vi "GameToIAStateOffensive.vi"(8 "error in (no error)":errorcluster, 11 "Game in":refnum<class "Game.lvclass">) -> (0 "error out":errorcluster, 1 "RobotRef":refnum<class "Robot.lvclass">[](array[class]), 2 "IA State out":T1={"our_robots"=[], "enemy_robots"=[], "balls"=[], "geometry"={"line_width"=0, "field_length"=0, "field_width"=0, "boundary_width"=0, "referee_width"=0, "goal_width"=0, "goal_depth"=0, "goal_wall_width"=0, "center_circle_radius"=0, "defense_radius"=0, "defense_stretch"=0, "free_kick_from_defense_dist"=0, "penalty_spot_from_field_line_dist"=0, "penalty_line_from_spot_dist"=0}, "IA Judge"={"stage"="", "command"="", "our_goalie_id"=0.0, "enemy_goalie_id"=0.0, "command enum"=enum."Halt", "Time"=enum."Azul"}, "Received Timestamp"=timestamp(0 s since 1904-01-01), "Events"={"Touch"=FALSE, "Ball out"=FALSE, "id touch"=0.0, "Ball out of \nVision"=FALSE, "Ball inside \nGoalie area"=FALSE, "Robot not responding"=FALSE, "Robots responding status"=[1.0, 1.0, 1.0, 1.0, 1.0, 1.0], "Enemy Ball \nPossession"=FALSE, "Pass State"=FALSE, "id end of pass"=0.0, "Kick"=FALSE, "Id ini Possession"=0.0, "Ball Possesion"=FALSE, "Id Possesion"=0.0, "Direct Kick"=FALSE, "2nd Strk Ativo"=FALSE}}, 3 "Game out":refnum<class "Game.lvclass">, 4 "Parameters.lvclass":refnum<class "Parameters.lvclass">)   [LabVIEW 2023, in "Game.lvclass"]
uses:
  Game.lvclass
  Vision_class/Old vision/SSL Detection Frame Simple Estimator Cameras VelCmd Folder/Core/AI Input.ctl
  Vision_class/Old vision/Controls/AI Robot.ctl
  Vision_class/Old vision/Controls/Functions Enum.ctl
  Vision_class/Old vision/Controls/AttackerStates.ctl
  Vision_class/Old vision/Controls/PathDests.ctl
  Vision_class/Old vision/Controls/PathDest.ctl
  Navigation/VSSNavigation/VSSAttackerStates.ctl
  Vision_class/Old vision/SSL Detection Frame Simple Estimator Cameras VelCmd Folder/Core/AI Ball.ctl
  Vision_class/Old vision/SSL Detection Frame Simple Estimator Cameras VelCmd Folder/Core/Field Size.ctl
  Vision_class/Old vision/SSL Detection Frame Simple Estimator Cameras VelCmd Folder/Core/AI Judge.ctl
  Communication_class/Paths/MessageAI_State Folder/Intel/Command Enum.ctl
  Vision_class/Old vision/SSL Detection Frame Simple Estimator Cameras VelCmd Folder/Util/Events/Events.ctl
  Robot_class/Robot.lvclass
  Parameters_class/Parameters.lvclass
  Team_class/OffensivePlay.ctl
  Game.lvclass/Game.ctl
  Team_class/Team.lvclass/Team.ctl
  Object_class/Object.lvclass/Object.ctl
  Ball_class/Ball.lvclass/Ball.ctl
  Events_class/Events.lvclass/Events.ctl
  Referee_class/Referee.lvclass/Referee.ctl
  Robot_class/Robot.lvclass/Robot.ctl
  Robot_class/Read id.vi
  Object_class/Read x.vi
  Object_class/Read y.vi
  Robot_class/Read orientation.vi
  Robot_class/Read est_v_tang.vi
  Robot_class/Read est_v_norm.vi
  Object_class/Read pos_est_x.vi
  Object_class/Read pos_est_y.vi
  Robot_class/Read dribble.vi
  Robot_class/Read path.vi
  Robot_class/Read path_smooth.vi
  Robot_class/Read dest_x.vi
  Robot_class/Read dest_y.vi
  Robot_class/Read dest_orientation.vi
  Robot_class/Read role.vi
  Read Parameters.lvclass.vi
  Read OffensiveTeam.vi
  Read EnemyRef.vi
  Read BallRef.vi
  Read EventsRef.vi
  Read FieldRef.vi
  Read Referee.vi
  Read TimeRef.vi
  Referee_class/Read command_from_referee.vi
  Referee_class/Read command_interpreted.vi
  Events_class/Read ball_inside_enemy_goalie_area.vi
  Events_class/Read ball_inside_our_goalie_area.vi
  Events_class/Read ball_out.vi
  Events_class/Read ball_out_of_vision.vi
  Events_class/Read enemy_ball_possesion.vi
  Events_class/Read id_enemy_ball_possesion.vi
  Events_class/Read id_our_balll_possesion.vi
  Events_class/Read id_touch.vi
  Events_class/Read kick.vi
  Events_class/Read our_balll_possesion.vi
  Events_class/Read touch.vi
  Ball_class/Read v_x.vi
  Ball_class/Read v_y.vi
  Team_class/Read RobotRef.vi
  Team_class/Read OffensivePlay.vi
  Ball_class/Ball.lvclass
  Enemy_class/Enemy.lvclass
  Ally_class/Ally.lvclass
  Events_class/Events.lvclass
  Field_class/Field.lvclass
  Referee_class/Referee.lvclass
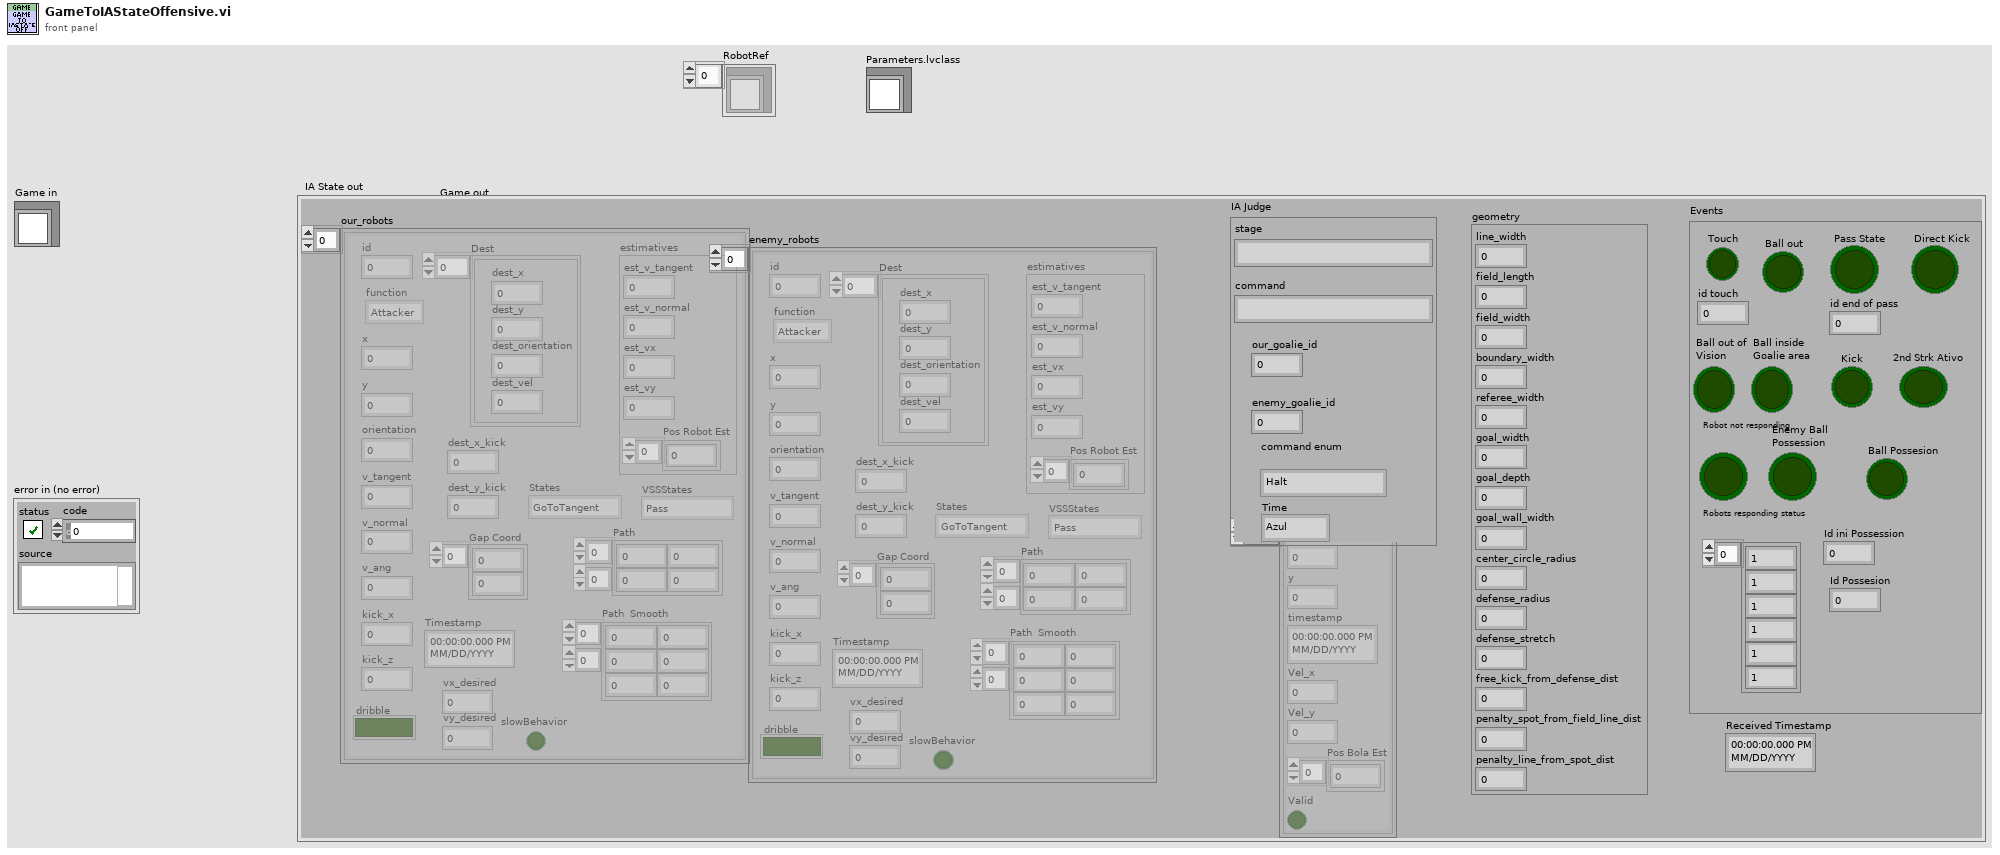
[diagram p1: front panel]
types:
  T1 = typedef "AI Input.ctl" = cluster{"our_robots":T2[], "enemy_robots":T2[], "balls":T8[], "geometry":T9, "IA Judge":T10, "Received Timestamp":timestamp, "Events":T12}
  T2 = typedef "AI Robot.ctl" = cluster{"id":u32, "function":T3, "x":dbl, "y":dbl, "orientation":dbl, "v_tangent":dbl, "v_normal":dbl, "v_ang":dbl, "kick_x":dbl, "kick_z":dbl, "dribble":bool, "Timestamp":timestamp, "estimatives":cluster{"est_v_tangent":dbl, "est_v_normal":dbl, "est_vx":dbl, "est_vy":dbl, "Pos Robot Est":dbl[]}, "dest_x_kick":dbl, "dest_y_kick":dbl, "Gap Coord":dbl[], "States":T4, "Path ":dbl[][], "Path  Smooth":dbl[][], "Dest":T5, "vx_desired":dbl, "vy_desired":dbl, "slowBehavior":bool, "VSSStates":T7}
  T3 = typedef "Functions Enum.ctl" = enum16{"2nd Striker", "Attacker", "Goalie", "Defender", "Striker", "Goto 0", "Dummy", "Kicker", "ZigZag 0", "ZigZag 1", "ZigZag 2", "ZigZag 3", "ZigZag 4", "ZigZag 5", "ZigZag 6", "ZigZag 7", "ZigZag 8", ""}
  T4 = typedef "AttackerStates.ctl" = enum16{"Pass", "GoToTangent", "BallGetting", "GoToKick", ""}
  T5 = typedef "PathDests.ctl" = T6[]
  T6 = typedef "PathDest.ctl" = cluster{"dest_x":dbl, "dest_y":dbl, "dest_orientation":dbl, "dest_vel":dbl}
  T7 = typedef "VSSAttackerStates.ctl" = enum16{"Pass", "GoToTangent", "BallGetting", "GoToKick", "Rotate anti-clockwise", "Rotate Clockwise", ""}
  T8 = typedef "AI Ball.ctl" = cluster{"x":dbl, "y":dbl, "timestamp":timestamp, "Vel_x":dbl, "Vel_y":dbl, "Pos Bola Est":dbl[], "Valid":bool}
  T9 = typedef "Field Size.ctl" = cluster{"line_width":u32, "field_length":u32, "field_width":u32, "boundary_width":u32, "referee_width":u32, "goal_width":u32, "goal_depth":u32, "goal_wall_width":u32, "center_circle_radius":u32, "defense_radius":u32, "defense_stretch":u32, "free_kick_from_defense_dist":u32, "penalty_spot_from_field_line_dist":u32, "penalty_line_from_spot_dist":u32}
  T10 = typedef "AI Judge.ctl" = cluster{"stage":string, "command":string, "our_goalie_id":dbl, "enemy_goalie_id":dbl, "command enum":T11, "Time":enum16{"Azul", "Amarelo"}}
  T11 = typedef "Command Enum.ctl" = enum16{"Halt", "Stop", "Force Start", "PKA Normal Start", "Prepare Kickoff Ally", "PKE Normal Start", "Prepare Kickoff Enemy", "Prepare Penalty Ally", "PPA Normal Start", "Prepare Penalty Enemy", "PPE Normal Start", "Direct Free Enemy", "Direct Free Ally", "Indirect Free Enemy", "Indirect Free Ally", "Timeout Enemy", "Timeout Ally", "Goal Enemy", "Goal Ally", "Ball Placement Enemy", "Ball Placement Ally", "Normal Half Time", "Extra Time Break", "Extra Half Time", "None", "Post Game"}
  T12 = typedef "Events.ctl" = cluster{"Touch":bool, "Ball out":bool, "id touch":dbl, "Ball out of \nVision":bool, "Ball inside \nGoalie area":bool, "Robot not responding":bool, "Robots responding status":dbl[], "Enemy Ball \nPossession":bool, "Pass State":bool, "id end of pass":dbl, "Kick":bool, "Id ini Possession":dbl, "Ball Possesion":bool, "Id Possesion":dbl, "Direct Kick":bool, "2nd Strk Ativo":bool}
  T13 = typedef "OffensivePlay.ctl" = enum16{"TableWithStriker", "TableWith2ndStrikerPlay", "PrepareDoublePass", "PrepareRollToPass", "SimplePass", "PreparePass", "PassToStriker", "BallOutOfField", "PassTo2ndStriker", "StopOffensive", "Prepare Penalty Enemy", "EnemyPossessionAtEnemyField", "EnemyPossesionAtOurField", "TestPlay", "PreparePenaltyAlly", "KickPenaltyAlly", "PrepareKickoffAlly", "PrepareKickoffEnemy", "IndirectEnemy", "DirectEnemy", "NormalGame", "DirectKick", "Pass", "Halt", "Timeout", "PassPlay", "PenaltyEnemy"}
  T14 = typedef "command_interpreted.ctl" = enum16{"Goal Ally", "Goal Enemy", "Ball Placement Enemy", "Ball Placement Ally", "Normal Half Time", "Extra Time  Break", "Extra Half Time", "None", "Post Game", "PKA Normal Start", "Prepare Kickoff Ally", "PKE Normal Start", "Prepare Kickoff Enemy", "Force Start", "Halt", "Timeout", "Prepare Penalty Ally", "Prepare Penalty Enemy", "PPA NormalStart", "PPE Normal Start", "Indirect Free Ally", "Direct Free Enemy", "Direct Free Ally", "Indirect Free Enemy", "Stop"}
  T15 = typedef "roles.ctl" = enum16{"BallChallengerAttackerVSS", "NormalAttackerVSS", "AttackerAimGoalVSS", "DefenderAreaVSS", "KeeperVSS", "Tabler", "TableFinalizer", "PrepareRollToPassRoller", "PrepareRollToPassReceiver", "SimplePassRoll", "SimplePassRollReceiver", "PenaltyDefense", "PreparePassReceiver 2", "PreparePassReceiver 1", "PassObserver", "Timeout", "Goto", "ZigZag", "None", "BallOutOfField", "DefenderArea", "Duelist", "AttackerStop", "FollowAttacker", "KeeperRole", "KickPenalty", "AttackerAimGoal", "AttackerBlock", "Marker", "Halt", "Shoot", "PassKicker", "PassReceiver", "TestRole", "PenaltyAttacker"}
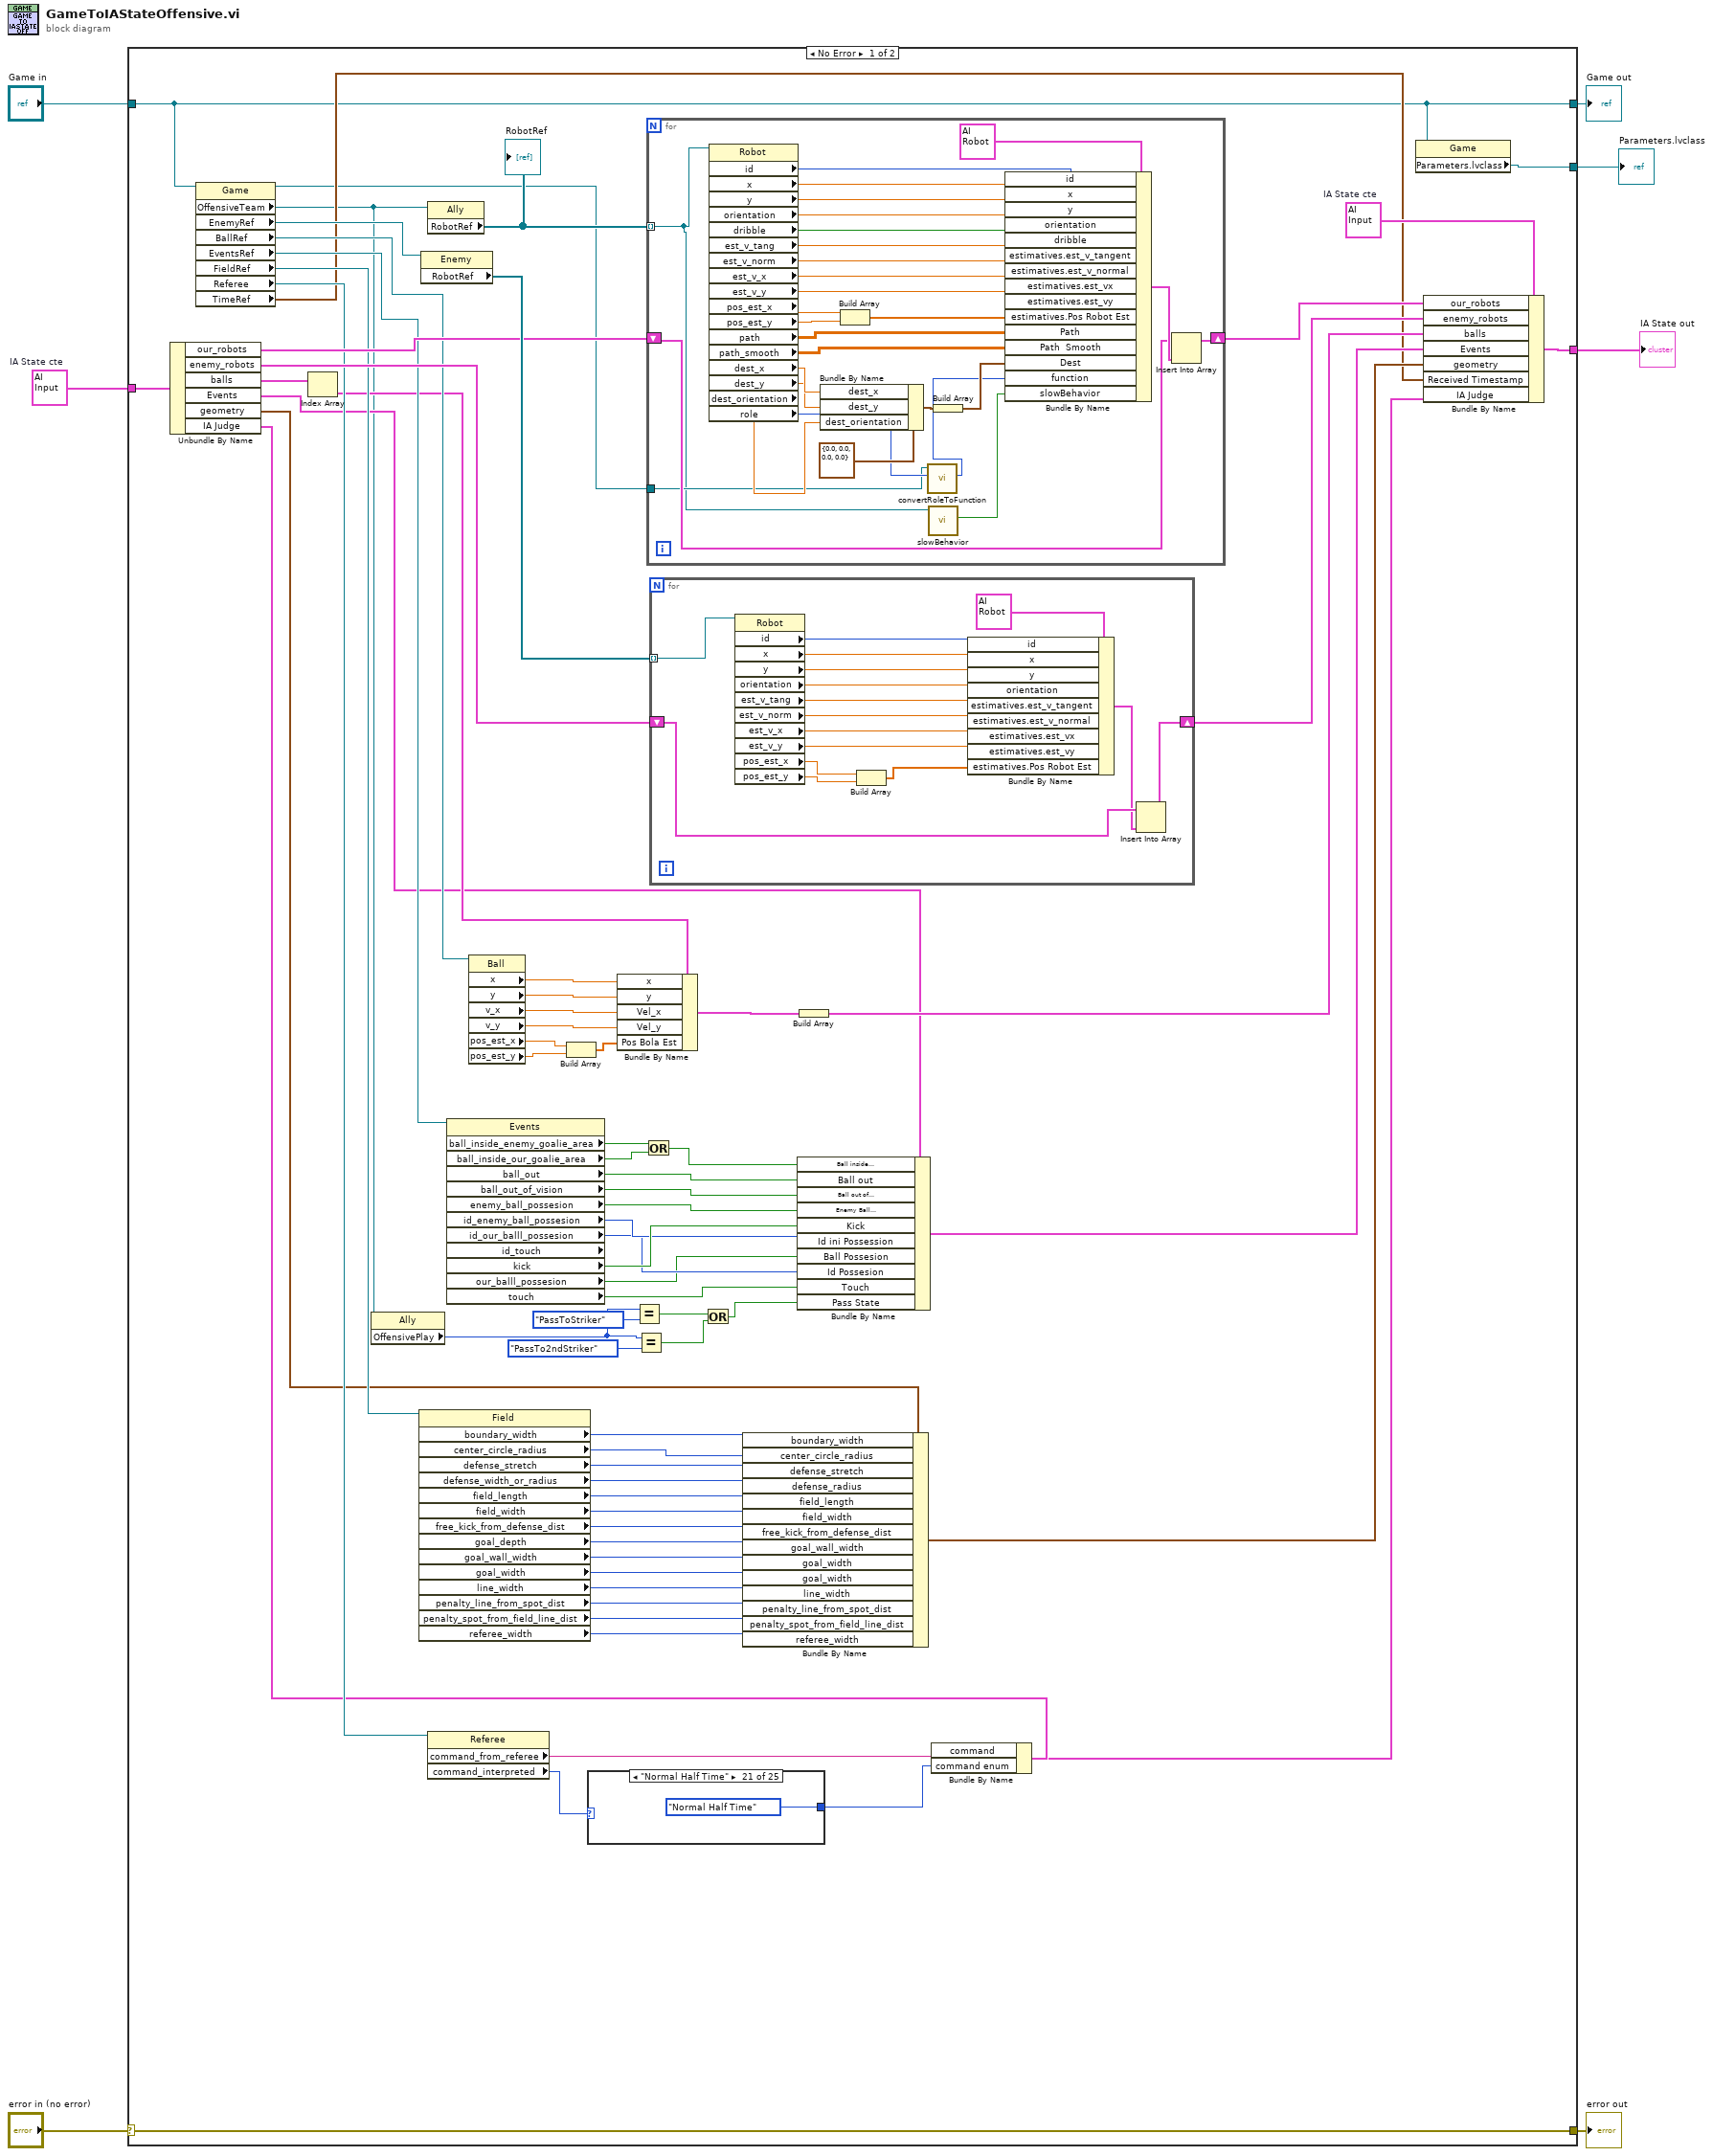
[diagram p0: block diagram]
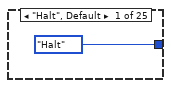
[diagram p2: hidden frame]
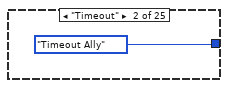
[diagram p3: hidden frame]
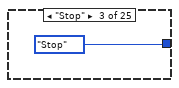
[diagram p4: hidden frame]
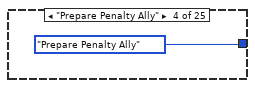
[diagram p5: hidden frame]
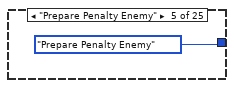
[diagram p6: hidden frame]
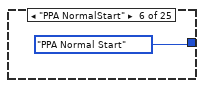
[diagram p7: hidden frame]
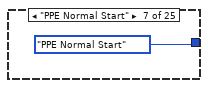
[diagram p8: hidden frame]
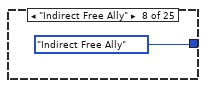
[diagram p9: hidden frame]
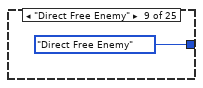
[diagram p10: hidden frame]
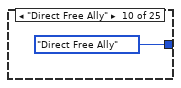
[diagram p11: hidden frame]
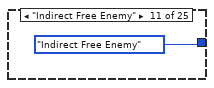
[diagram p12: hidden frame]
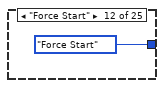
[diagram p13: hidden frame]
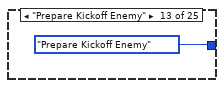
[diagram p14: hidden frame]
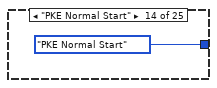
[diagram p15: hidden frame]
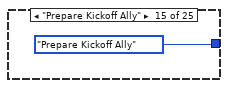
[diagram p16: hidden frame]
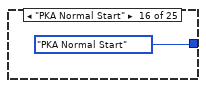
[diagram p17: hidden frame]
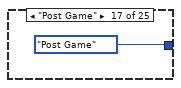
[diagram p18: hidden frame]
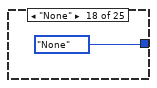
[diagram p19: hidden frame]
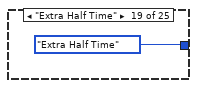
[diagram p20: hidden frame]
diagram:
  w3 = T1 {"our_robots"=[], "enemy_robots"=[], "balls"=[], "geometry"={"line_width"=0, "field_length"=0, "field_width"=0, "boundary_width"=0, "referee_width"=0, "goal_width"=0, "goal_depth"=0, "goal_wall_width"=0, "center_circle_radius"=0, "defense_radius"=0, "defense_stretch"=0, "free_kick_from_defense_dist"=0, "penalty_spot_from_field_line_dist"=0, "penalty_line_from_spot_dist"=0}, "IA Judge"={"stage"="", "command"="", "our_goalie_id"=0.0, "enemy_goalie_id"=0.0, "command enum"=enum."Halt", "Time"=enum."Azul"}, "Received Timestamp"=timestamp(0 s since 1904-01-01), "Events"={"Touch"=FALSE, "Ball out"=FALSE, "id touch"=0.0, "Ball out of \nVision"=FALSE, "Ball inside \nGoalie area"=FALSE, "Robot not responding"=FALSE, "Robots responding status"=[], "Enemy Ball \nPossession"=FALSE, "Pass State"=FALSE, "id end of pass"=0.0, "Kick"=FALSE, "Id ini Possession"=0.0, "Ball Possesion"=FALSE, "Id Possesion"=0.0, "Direct Kick"=FALSE, "2nd Strk Ativo"=FALSE}}  # IA State cte
  n1 = case shown="No Error" "error in (no error)" {
    selector: "error in (no error)" -> [w78 w151]
    tunnel: [w78 w151] -> w6
    tunnel: [w9 w150] -> w4
    tunnel: "Game in" -> [w9 w150]
    tunnel: w3 -> [w74 w149]
    tunnel: [w18 w149] -> w2
    tunnel: [w8 _] -> w1
    frame No Error {
      w70 = T1 {"our_robots"=[], "enemy_robots"=[], "balls"=[], "geometry"={"line_width"=0, "field_length"=0, "field_width"=0, "boundary_width"=0, "referee_width"=0, "goal_width"=0, "goal_depth"=0, "goal_wall_width"=0, "center_circle_radius"=0, "defense_radius"=0, "defense_stretch"=0, "free_kick_from_defense_dist"=0, "penalty_spot_from_field_line_dist"=0, "penalty_line_from_spot_dist"=0}, "IA Judge"={"stage"="", "command"="", "our_goalie_id"=0.0, "enemy_goalie_id"=0.0, "command enum"=enum."Halt", "Time"=enum."Azul"}, "Received Timestamp"=timestamp(0 s since 1904-01-01), "Events"={"Touch"=FALSE, "Ball out"=FALSE, "id touch"=0.0, "Ball out of \nVision"=FALSE, "Ball inside \nGoalie area"=FALSE, "Robot not responding"=FALSE, "Robots responding status"=[], "Enemy Ball \nPossession"=FALSE, "Pass State"=FALSE, "id end of pass"=0.0, "Kick"=FALSE, "Id ini Possession"=0.0, "Ball Possesion"=FALSE, "Id Possesion"=0.0, "Direct Kick"=FALSE, "2nd Strk Ativo"=FALSE}}  # IA State cte
      n2 = Unbundle By Name(w74) -> ("our_robots"=w73:T2[], "enemy_robots"=w72:T2[], "balls"=w27:T8[], "Events"=w25:T12, "geometry"=w24:T9, "IA Judge"=w22:T10)
      n3 = property class="Game"(reference=w9) -> (reference out=w10:refnum<class "Game.lvclass">, "OffensiveTeam"=w17:refnum<class "Ally.lvclass">, "EnemyRef"=w76:refnum<class "Enemy.lvclass">, "BallRef"=w71:refnum<class "Ball.lvclass">, "EventsRef"=w58:refnum<class "Events.lvclass">, "FieldRef"=w45:refnum<class "Field.lvclass">, "Referee"=w29:refnum<class "Referee.lvclass">, "TimeRef"=w23:timestamp)  [unwired: 1 in, 1 out]
      n4 = Index Array(array=w27) -> (element=w26:T8)  [unwired: 1 in]
      n5 = property class="Ally"(reference=w17) -> ("OffensivePlay"=w13:T13)  [unwired: 1 in, 2 out]
      n6 = property class="Field"(reference=w45) -> ("boundary_width"=w44:i32, "center_circle_radius"=w43:i32, "defense_stretch"=w42:i32, "defense_width_or_radius"=w41:i32, "field_length"=w40:i32, "field_width"=w39:i32, "free_kick_from_defense_dist"=w38:i32, "goal_depth"=w37:i32, "goal_wall_width"=w36:i32, "goal_width"=w35:i32, "line_width"=w34:i32, "penalty_line_from_spot_dist"=w33:i32, "penalty_spot_from_field_line_dist"=w32:i32, "referee_width"=w31:i32)  [unwired: 1 in, 2 out]
      n7 = property class="Enemy"(reference=w76) -> ("RobotRef"=w75:refnum<class "Robot.lvclass">[])  [unwired: 1 in, 2 out]
      n8 = property class="Ally"(reference=w17) -> ("RobotRef"=w77:refnum<class "Robot.lvclass">[])  [unwired: 1 in, 2 out]
      "RobotRef" <- w77
      n9 = property class="Referee"(reference=w29) -> ("command_from_referee"=w28:string, "command_interpreted"=w21:T14)  [unwired: 1 in, 2 out]
      n10 = property class="Events" props=["ball_inside_enemy_goalie_area", "ball_inside_our_goalie_area", "ball_out", "ball_out_of_vision", "enemy_ball_possesion", "id_enemy_ball_possesion", "id_our_balll_possesion", "id_touch", "kick", "our_balll_possesion", "touch"](reference=w58) -> ("ball_inside_enemy_goalie_area"=w56:bool, "ball_inside_our_goalie_area"=w57:bool, "ball_out"=w54:bool, "ball_out_of_vision"=w53:bool, "enemy_ball_possesion"=w52:bool, "id_enemy_ball_possesion"=w50:i32, "id_our_balll_possesion"=w49:i32, "kick"=w51:bool, "our_balll_possesion"=w48:bool, "touch"=w47:bool)  [unwired: 1 in, 3 out]
      n11 = property class="Ball"(reference=w71) -> ("x"=w67:dbl, "y"=w66:dbl, "v_x"=w65:dbl, "v_y"=w64:dbl, "pos_est_x"=w63:dbl, "pos_est_y"=w62:dbl)  [unwired: 1 in, 2 out]
      n12 = Build Array(w63, w62) -> (w61:dbl[])
      n13 = case shown="\"Normal Half Time\"" w21 {
        tunnel: [Command_Enum."Halt" ("command enum") Command_Enum."Timeout Ally" ("command enum") Command_Enum."Stop" ("command enum") Command_Enum."Prepare Penalty Ally" ("command enum") Command_Enum."Prepare Penalty Enemy" ("command enum") Command_Enum."PPA Normal Start" ("command enum") Command_Enum."PPE Normal Start" ("command enum") Command_Enum."Indirect Free Ally" ("command enum") Command_Enum."Direct Free Enemy" ("command enum") Command_Enum."Direct Free Ally" ("command enum") Command_Enum."Indirect Free Enemy" ("command enum") Command_Enum."Force Start" ("command enum") Command_Enum."Prepare Kickoff Enemy" ("command enum") Command_Enum."PKE Normal Start" ("command enum") Command_Enum."Prepare Kickoff Ally" ("command enum") Command_Enum."PKA Normal Start" ("command enum") Command_Enum."Post Game" ("command enum") Command_Enum."None" ("command enum") Command_Enum."Extra Half Time" ("command enum") Command_Enum."Extra Time Break" ("command enum") Command_Enum."Normal Half Time" ("command enum") Command_Enum."Ball Placement Ally" ("command enum") Command_Enum."Ball Placement Enemy" ("command enum") Command_Enum."Goal Enemy" ("command enum") Command_Enum."Goal Ally" ("command enum")] -> w20
        frame "Halt", Default {
        }
        frame "Timeout" {
        }
        frame "Stop" {
        }
        frame "Prepare Penalty Ally" {
        }
        frame "Prepare Penalty Enemy" {
        }
        frame "PPA NormalStart" {
        }
        frame "PPE Normal Start" {
        }
        frame "Indirect Free Ally" {
        }
        frame "Direct Free Enemy" {
        }
        frame "Direct Free Ally" {
        }
        frame "Indirect Free Enemy" {
        }
        frame "Force Start" {
        }
        frame "Prepare Kickoff Enemy" {
        }
        frame "PKE Normal Start" {
        }
        frame "Prepare Kickoff Ally" {
        }
        frame "PKA Normal Start" {
        }
        frame "Post Game" {
        }
        frame "None" {
        }
        frame "Extra Half Time" {
        }
        frame "Extra Time  Break" {
        }
        frame "Normal Half Time" {
        }
        frame "Ball Placement Ally" {
        }
        frame "Ball Placement Enemy" {
        }
        frame "Goal Enemy" {
        }
        frame "Goal Ally" {
        }
      }
      n14 = Bundle By Name(cluster=w26, "x"=w67, "y"=w66, "Vel_x"=w65, "Vel_y"=w64, "Pos Bola Est"=w61) -> (w60:T8)
      n15 = Equal?(x=w13, y=OffensivePlay."PassToStriker") -> (x = y?=w15:bool)
      n16 = Equal?(x=w13, y=OffensivePlay."PassTo2ndStriker") -> (x = y?=w12:bool)
      n17 = Or(x=w56, y=w57) -> (x .or. y?=w55:bool)
      n18 = for {
        tunnel: w77 -> [w105] mode=indexing
        shift-right: [w129] -> w69
        shift-left: w73 -> [w130]
        tunnel: w10 -> [w106]
        n19 = property class="Robot"(reference=w105) -> ("id"=w128:i32, "x"=w127:dbl, "y"=w126:dbl, "orientation"=w125:dbl, "dribble"=w124:bool, "est_v_tang"=w123:dbl, "est_v_norm"=w122:dbl, "est_v_x"=w121:dbl, "est_v_y"=w120:dbl, "pos_est_x"=w119:dbl, "pos_est_y"=w118:dbl, "path"=w116:dbl[][], "path_smooth"=w115:dbl[][], "dest_x"=w114:dbl, "dest_y"=w113:dbl, "dest_orientation"=w112:dbl, "role"=w108:T15)  [unwired: 1 in, 2 out]
        n20 = Bundle By Name(cluster=T6 {"dest_x"=0.0, "dest_y"=0.0, "dest_orientation"=0.0, "dest_vel"=0.0} ("element"), "dest_x"=w114, "dest_y"=w113, "dest_orientation"=w112) -> (w110:T6)
        n21 = Build Array(w119, w118) -> (w117:dbl[])
        n22 = call "convertRoleToFunction.vi"("role"=w108, "Game in"=w106) -> ("function"=w107:T3)  [unwired: 7 in, 2 out]
        n23 = call "slowBehavior.vi"("Robot in"=w105) -> ("slowBehabior"=w104:bool)  [unwired: 8 in, 2 out]
        n24 = Build Array(w110) -> (w109:T6[])
        n25 = Bundle By Name(cluster=T2 {"id"=0, "function"=enum."Attacker", "x"=0.0, "y"=0.0, "orientation"=0.0, "v_tangent"=0.0, "v_normal"=0.0, "v_ang"=0.0, "kick_x"=0.0, "kick_z"=0.0, "dribble"=FALSE, "Timestamp"=timestamp(0 s since 1904-01-01), "estimatives"={"est_v_tangent"=0.0, "est_v_normal"=0.0, "est_vx"=0.0, "est_vy"=0.0, "Pos Robot Est"=[]}, "dest_x_kick"=0.0, "dest_y_kick"=0.0, "Gap Coord"=[], "States"=enum."GoToTangent", "Path "=[], "Path  Smooth"=[], "Dest"=[], "vx_desired"=0.0, "vy_desired"=0.0, "slowBehavior"=FALSE, "VSSStates"=enum."Pass"} ("Robot"), "id"=w128, "x"=w127, "y"=w126, "orientation"=w125, "dribble"=w124, "estimatives.est_v_tangent"=w123, "estimatives.est_v_normal"=w122, "estimatives.est_vx"=w121, "estimatives.est_vy"=w120, "estimatives.Pos Robot Est"=w117, "Path"=w116, "Path  Smooth"=w115, "Dest"=w109, "function"=w107, "slowBehavior"=w104) -> (w131:T2)
        n26 = Insert Into Array(array=w130, new element=w131) -> (w129:T2[])  [unwired: 1 in]
      }
      n27 = for {
        tunnel: w75 -> [w143] mode=indexing
        shift-right: [w133] -> w68
        shift-left: w72 -> [w142]
        n28 = property class="Robot"(reference=w143) -> ("id"=w145:i32, "x"=w146:dbl, "y"=w147:dbl, "orientation"=w148:dbl, "est_v_tang"=w141:dbl, "est_v_norm"=w140:dbl, "est_v_x"=w139:dbl, "est_v_y"=w138:dbl, "pos_est_x"=w137:dbl, "pos_est_y"=w136:dbl)  [unwired: 1 in, 2 out]
        n29 = Build Array(w137, w136) -> (w135:dbl[])
        n30 = Bundle By Name(cluster=T2 {"id"=0, "function"=enum."Attacker", "x"=0.0, "y"=0.0, "orientation"=0.0, "v_tangent"=0.0, "v_normal"=0.0, "v_ang"=0.0, "kick_x"=0.0, "kick_z"=0.0, "dribble"=FALSE, "Timestamp"=timestamp(0 s since 1904-01-01), "estimatives"={"est_v_tangent"=0.0, "est_v_normal"=0.0, "est_vx"=0.0, "est_vy"=0.0, "Pos Robot Est"=[]}, "dest_x_kick"=0.0, "dest_y_kick"=0.0, "Gap Coord"=[], "States"=enum."GoToTangent", "Path "=[], "Path  Smooth"=[], "Dest"=[], "vx_desired"=0.0, "vy_desired"=0.0, "slowBehavior"=FALSE, "VSSStates"=enum."Pass"} ("Robot"), "id"=w145, "x"=w146, "y"=w147, "orientation"=w148, "estimatives.est_v_tangent"=w141, "estimatives.est_v_normal"=w140, "estimatives.est_vx"=w139, "estimatives.est_vy"=w138, "estimatives.Pos Robot Est"=w135) -> (w134:T2)
        n31 = Insert Into Array(array=w142, new element=w134) -> (w133:T2[])  [unwired: 1 in]
      }
      n32 = Or(x=w15, y=w12) -> (x .or. y?=w11:bool)
      n33 = Bundle By Name(cluster=w24, "boundary_width"=w44, "center_circle_radius"=w43, "defense_stretch"=w42, "defense_radius"=w41, "field_length"=w40, "field_width"=w39, "free_kick_from_defense_dist"=w38, "goal_wall_width"=w37, "goal_width"=w36, "goal_width"=w35, "line_width"=w34, "penalty_line_from_spot_dist"=w33, "penalty_spot_from_field_line_dist"=w32, "referee_width"=w31) -> (w30:T9)
      n34 = Bundle By Name(cluster=w25, "Ball inside \nGoalie area"=w55, "Ball out"=w54, "Ball out of \nVision"=w53, "Enemy Ball \nPossession"=w52, "Kick"=w51, "Id ini Possession"=w50, "Ball Possesion"=w48, "Id Possesion"=w49, "Touch"=w47, "Pass State"=w11) -> (w46:T12)
      n35 = Build Array(w60) -> (w59:T8[])
      n36 = Bundle By Name(cluster=w22, "command"=w28, "command enum"=w20) -> (w19:T10)
      n37 = property class="Game"(reference=w9) -> ("Parameters.lvclass"=w8:refnum<class "Parameters.lvclass">)  [unwired: 1 in, 2 out]
      n38 = Bundle By Name(cluster=w70, "our_robots"=w69, "enemy_robots"=w68, "balls"=w59, "Events"=w46, "geometry"=w30, "Received Timestamp"=w23, "IA Judge"=w19) -> (w18:T1)
    }
    frame Error {
    }
  }
  "error out" <- w6
  "Game out" <- w4
  "IA State out" <- w2
  "Parameters.lvclass" <- w1
